vi "Read TDMS_Report.vi"   [LabVIEW 2009]
doc: "This is a simple VI that calls the function which reads a TDMS file. For those who are not familiar with TDMS files using it will save them a few steps.\n\nAAL 9/09"
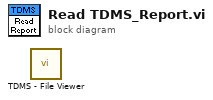
[diagram p0: block diagram]
diagram:
  n1 = call <vilib>:"TDMS - File Viewer.vi"() -> ()  [unwired: 2 in, 6 out]
